vi "FRAS Module.vi"(0 "Cluster DATA TCL-TCL":T1={"SF_Mode"=enum."Repos", "SF_8x1_donnees(t)"=[], "SF_dark_monopixels"=[], "SF_lambdas"=[0.0, 0.0], "SF_matrice_ABCD"=[[0.0, 0.0, 0.0, 0.0], [0.0, 0.0, 0.0, 0.0], [0.0, 0.0, 0.0, 0.0], [0.0, 0.0, 0.0, 0.0], [0.0, 0.0, 0.0, 0.0], [0.0, 0.0, 0.0, 0.0], [0.0, 0.0, 0.0, 0.0], [0.0, 0.0, 0.0, 0.0]], "SF_ref"=0.0, "SF_ref_mode"=enum."Repos", "SF_ref_fichier"=0.0, "SF_OPD_estime"=[0.0, 0.0], "SF_OPD_mesure"=[[0.0, 0.0]], "SF_OPD_residus"=[[0.0, 0.0]], "SF_OPD_commande"=0.0, "SF_Intensites"=[0.0, 0.0], "SF_variables"=[], "SF_gain_int"=0.0, "FRAS_Mode"=enum."Repos", "FRAS_image_a"=[], "FRAS_image_b"=[], "FRAS_ref_images"=[], "FRAS_ref_mode"=enum."Repos", "FRAS_ref_fichier"=[], "FRAS_taille_images"=0, "FRAS_pourcentage_seuil"=0.0, "FRAS_CdG_calibration"=FALSE, "FRAS_CdG(t)"=[], "FRAS_CdG(t+1)"=[], "FRAS_CdG_residus"=[], "FRAS_gain_int"=0.0, "PERT_Mode"=enum."Repos", "PERT_saut_frange"=0, "PERT_offset"=[0.0, 0.0], "PERT_rep_PI"=0.0, "Nb Repetitions"=32, "PERT_booléens"=[], "coefficients"=[], "matrice_commande"=[], "Commande"=[], "Stop"=FALSE, "Nb boucles"=0, "Nb Retards"=0, "Nb Echantillons"=32, "Sauvegarde"=FALSE, "Nb Echantillons Cam"=32, "Increment Dark"=32, "SF_v_mesure"=[0.0, 0.0], "NbRepetConsig"=0, "DimConsignExt"=0, "ConsignExt"=[], "SF_Ref'"=0.0, "FRAS_Ref'"=[]}, 7 "Nb boucle":i32, 11 "entree d'erreur":errorcluster) -> (4 "Cluster DATA TCL-TCL":T1={"SF_Mode"=enum."Repos", "SF_8x1_donnees(t)"=[], "SF_dark_monopixels"=[], "SF_lambdas"=[0.0, 0.0], "SF_matrice_ABCD"=[[0.0, 0.0, 0.0, 0.0], [0.0, 0.0, 0.0, 0.0], [0.0, 0.0, 0.0, 0.0], [0.0, 0.0, 0.0, 0.0], [0.0, 0.0, 0.0, 0.0], [0.0, 0.0, 0.0, 0.0], [0.0, 0.0, 0.0, 0.0], [0.0, 0.0, 0.0, 0.0]], "SF_ref"=0.0, "SF_ref_mode"=enum."Repos", "SF_ref_fichier"=0.0, "SF_OPD_estime"=[0.0, 0.0], "SF_OPD_mesure"=[[0.0, 0.0]], "SF_OPD_residus"=[[0.0, 0.0]], "SF_OPD_commande"=0.0, "SF_Intensites"=[0.0, 0.0], "SF_variables"=[], "SF_gain_int"=0.0, "FRAS_Mode"=enum."Repos", "FRAS_image_a"=[], "FRAS_image_b"=[], "FRAS_ref_images"=[], "FRAS_ref_mode"=enum."Repos", "FRAS_ref_fichier"=[], "FRAS_taille_images"=0, "FRAS_pourcentage_seuil"=0.0, "FRAS_CdG_calibration"=FALSE, "FRAS_CdG(t)"=[], "FRAS_CdG(t+1)"=[], "FRAS_CdG_residus"=[], "FRAS_gain_int"=0.0, "PERT_Mode"=enum."Repos", "PERT_saut_frange"=0, "PERT_offset"=[0.0, 0.0], "PERT_rep_PI"=0.0, "Nb Repetitions"=32, "PERT_booléens"=[], "coefficients"=[], "matrice_commande"=[], "Commande"=[], "Stop"=FALSE, "Nb boucles"=0, "Nb Retards"=0, "Nb Echantillons"=32, "Sauvegarde"=FALSE, "Nb Echantillons Cam"=32, "Increment Dark"=32, "SF_v_mesure"=[0.0, 0.0], "NbRepetConsig"=0, "DimConsignExt"=0, "ConsignExt"=[], "SF_Ref'"=0.0, "FRAS_Ref'"=[]}, 15 "sortie d'erreur 2":errorcluster caption="sortie d'erreur")   [LabVIEW 2020]
uses:
  ACCROCHAGE/XPS_FGV.ctl
  DATACluster.ctl
panel:
  out "FRAS_ref_fichier":sgl[][](array[numeric])
  out "FRAS_Ref'":dbl[][](array[numeric])
  out "SF_Ref'":dbl
  out "ConsignExtSF":dbl[](array[numeric])
  out "ConsignExtFRAS":dbl[](array[numeric])
  out "cluster de sortie":cluster{"OPD":dbl, "W":dbl, "v_est":dbl}
  out "v2":dbl
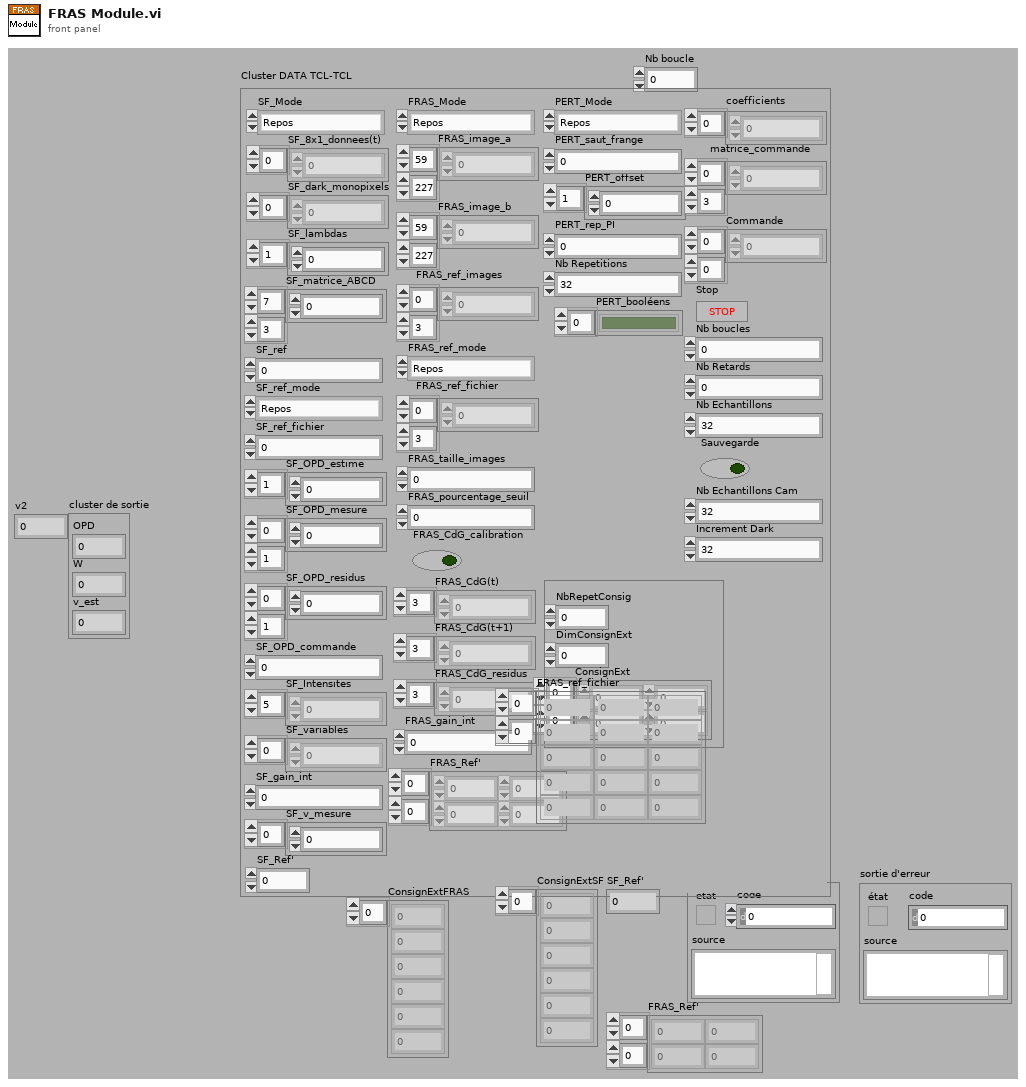
[diagram p1: front panel]
types:
  T1 = typedef "DATACluster.ctl" = cluster{"SF_Mode":enum16{"Repos", "Détection", "Acquisition", "Poursuite PID", "Poursuite Kalman", "Poursuite + contrôle"}, "SF_8x1_donnees(t)":dbl[], "SF_dark_monopixels":dbl[], "SF_lambdas":dbl[], "SF_matrice_ABCD":dbl[][], "SF_ref":dbl, "SF_ref_mode":enum16{"Repos", "Calibration", "Fichier"}, "SF_ref_fichier":dbl, "SF_OPD_estime":dbl[], "SF_OPD_mesure":dbl[][], "SF_OPD_residus":dbl[][], "SF_OPD_commande":dbl, "SF_Intensites":dbl[], "SF_variables":dbl[], "SF_gain_int":dbl, "FRAS_Mode":enum16{"Repos", "Détection", "Acquisition", "Poursuite", "Poursuite en a", "Poursuite en b"}, "FRAS_image_a":sgl[][], "FRAS_image_b":sgl[][], "FRAS_ref_images":sgl[][], "FRAS_ref_mode":enum16{"Repos", "Calibration", "Fichier"}, "FRAS_ref_fichier":sgl[][], "FRAS_taille_images":i32, "FRAS_pourcentage_seuil":sgl, "FRAS_CdG_calibration":bool, "FRAS_CdG(t)":dbl[], "FRAS_CdG(t+1)":dbl[], "FRAS_CdG_residus":dbl[], "FRAS_gain_int":dbl, "PERT_Mode":enum16{"Repos", "Calibration", "Fichier"}, "PERT_saut_frange":i8, "PERT_offset":dbl[], "PERT_rep_PI":dbl, "Nb Repetitions":i32, "PERT_booléens":bool[], "coefficients":dbl[], "matrice_commande":dbl[][], "Commande":dbl[][], "Stop":bool, "Nb boucles":i32, "Nb Retards":i16, "Nb Echantillons":i32, "Sauvegarde":bool, "Nb Echantillons Cam":i32, "Increment Dark":i32, "SF_v_mesure":dbl[], "NbRepetConsig":i32, "DimConsignExt":i32, "ConsignExt":dbl[][], "SF_Ref'":dbl, "FRAS_Ref'":dbl[][]}
  T2 = enum16{"Initialisation", "Acquisition", "Fermeture"}
  T3 = enum16{"Initialisation", "Calcul CdG a", "Calcul CdG b"}
  T4 = cluster{"Relative Target Position (units)":dbl, "Absolute Target Position (mm)":dbl}
  T5 = typedef "XPS_FGV.ctl" = enum16{"Init", "GroupKill", "GroupMotionEn", "GroupInit", "GroupHome", "ReadCurPos", "MoveAbs", "MoveRelatif", "JogEnable", "JogSet", "JogGet", "JogDisable", "ReadConfig", "GroupMotionDis", "Reboot", "Close"}
  T6 = cluster{"Velocity (units/s)":dbl, "Acceleration (units/s²)":dbl}
  T7 = typedef "IMAQ Image.ctl" = refnum<image>
  T8 = enum16{"Repos", "Détection", "Acquisition", "Poursuite", "Poursuite en a", "Poursuite en b"}
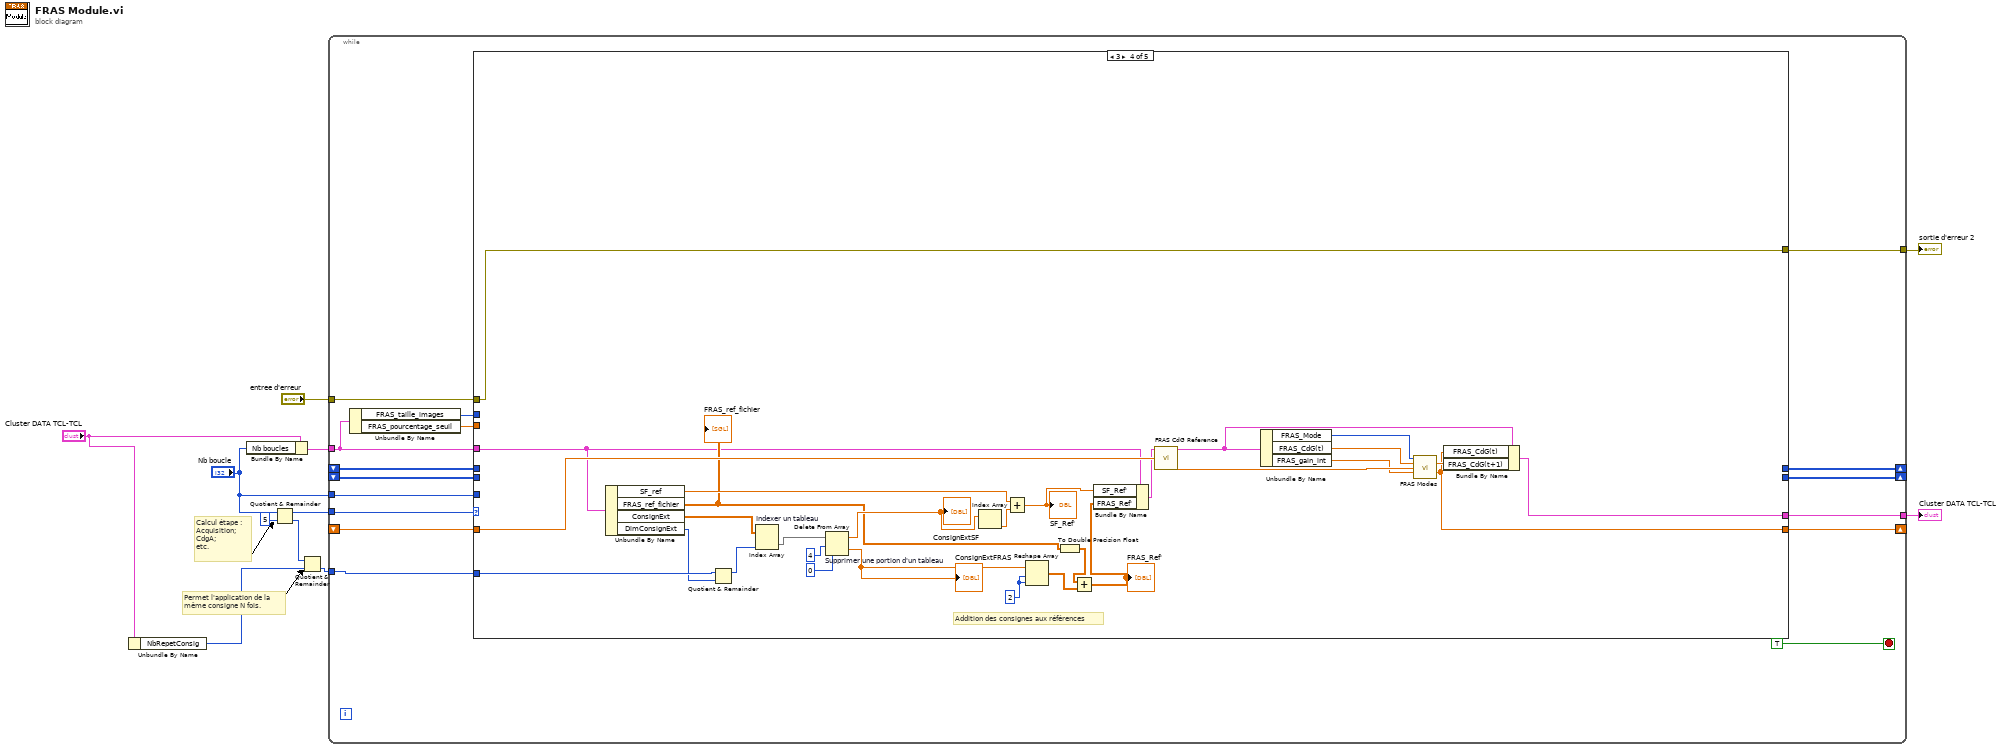
[diagram p0: block diagram]
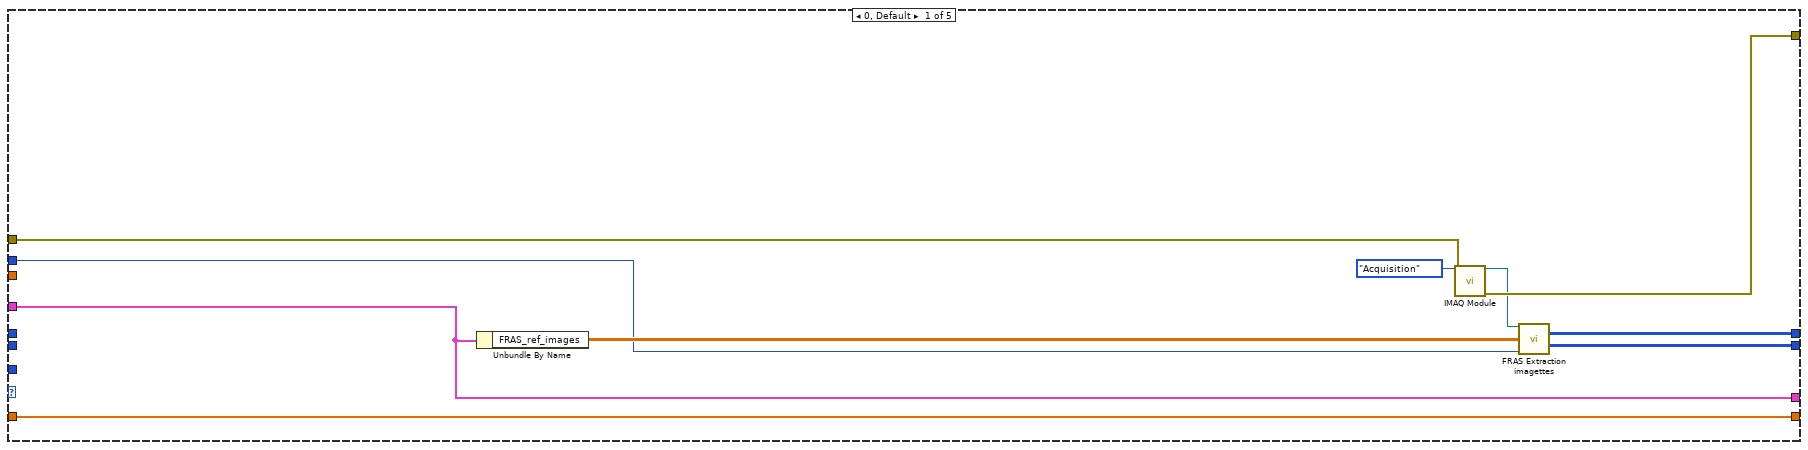
[diagram p2: hidden frame]
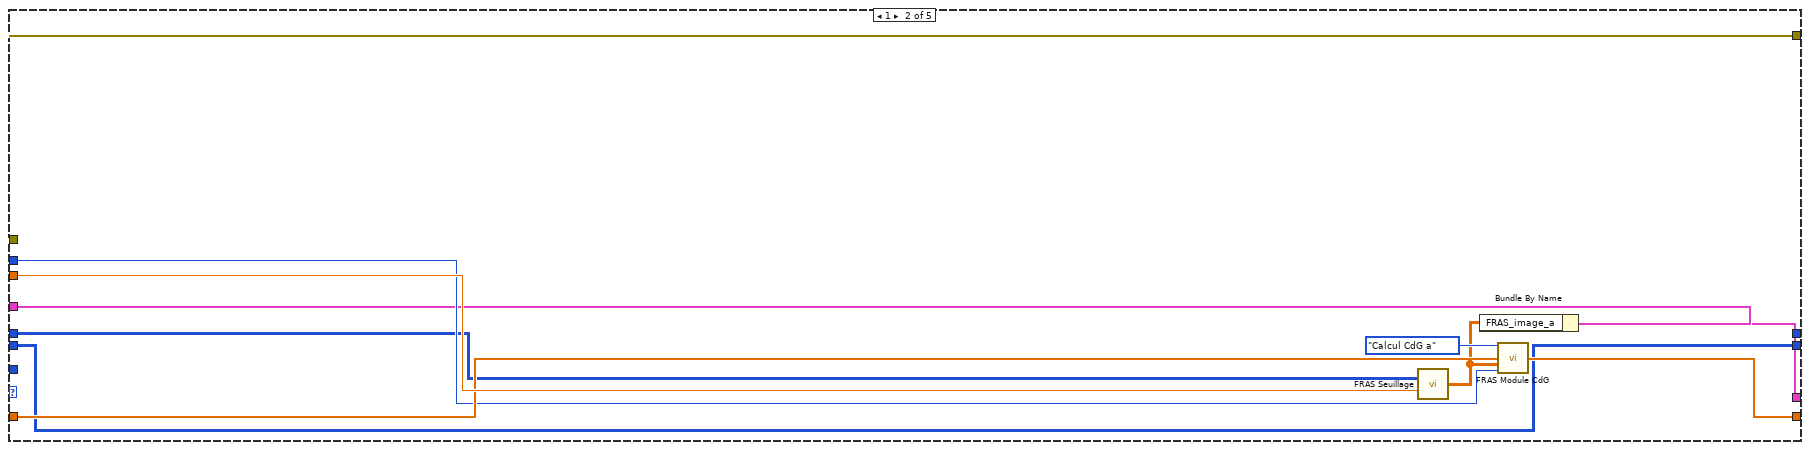
[diagram p3: hidden frame]
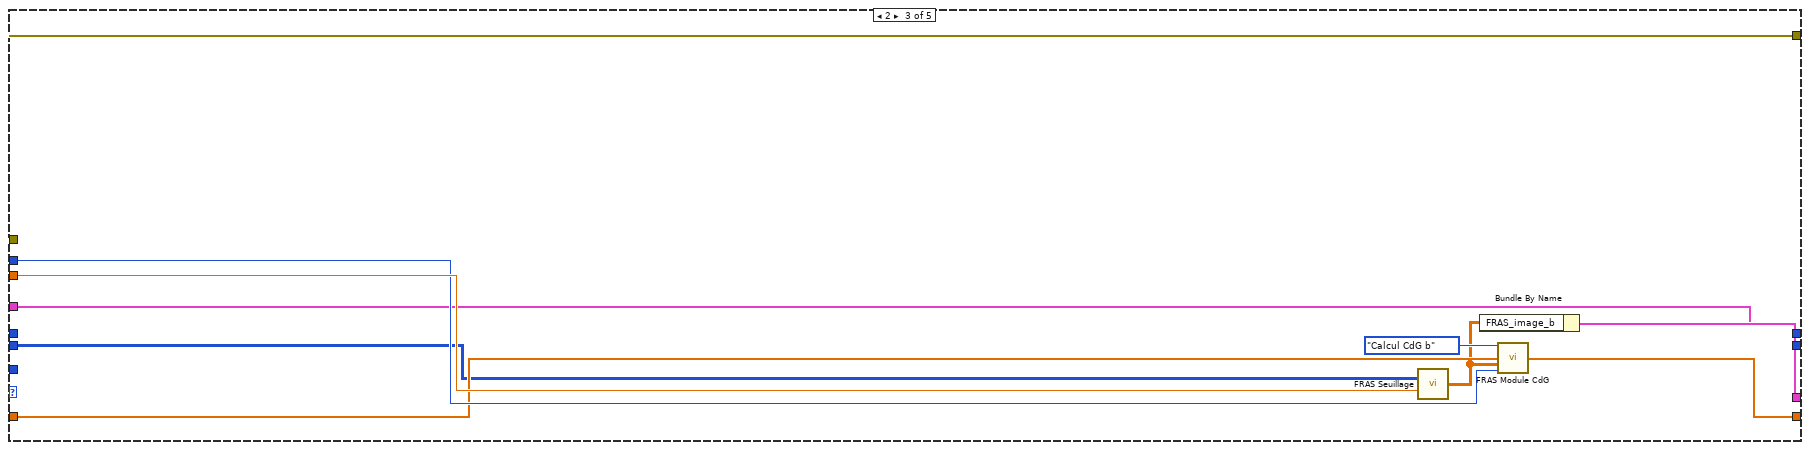
[diagram p4: hidden frame]
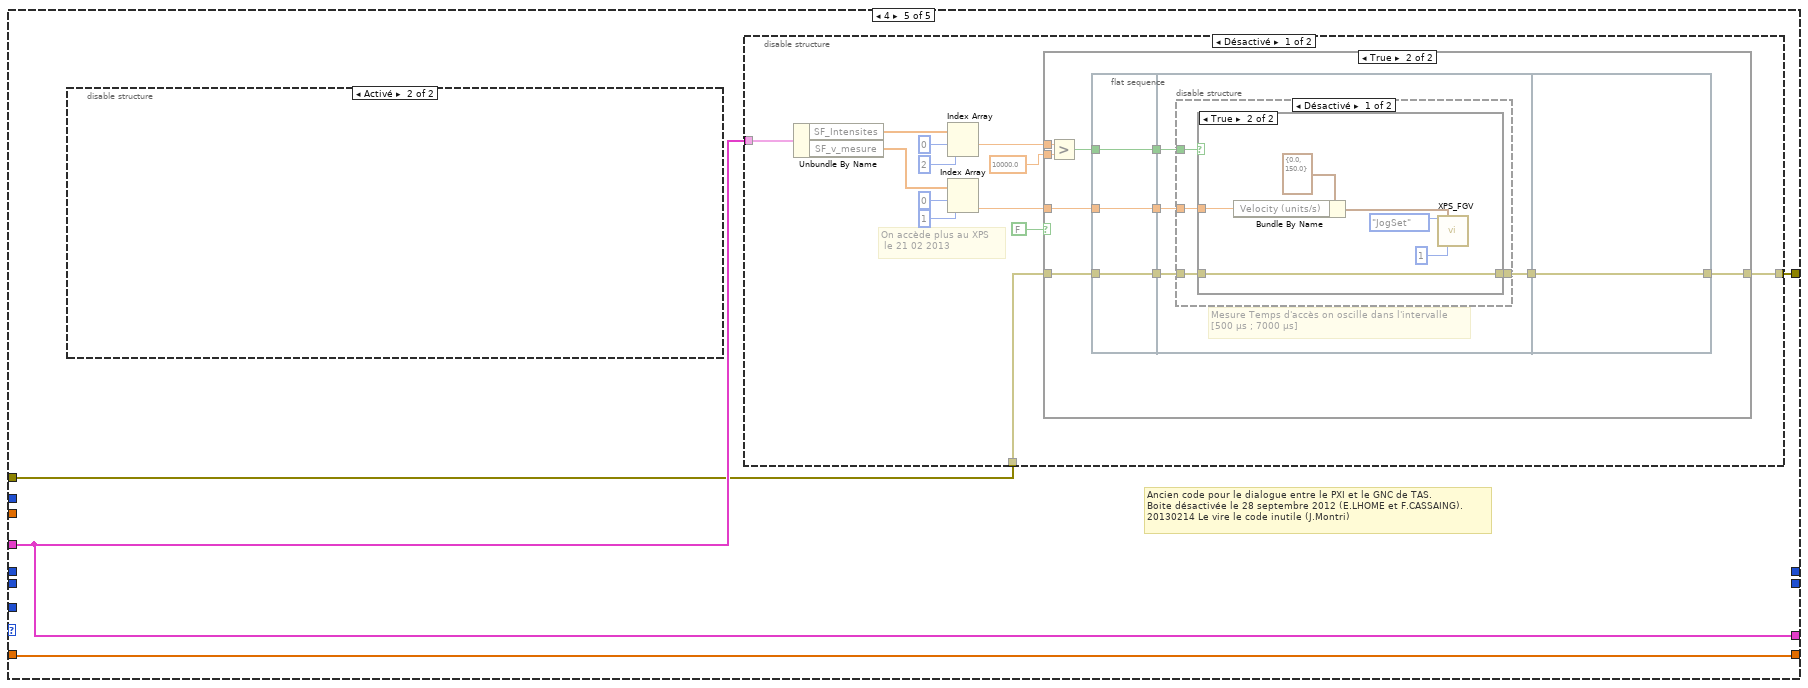
[diagram p5: hidden frame]
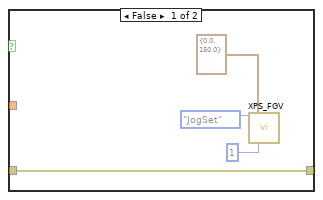
[diagram p7: hidden frame]
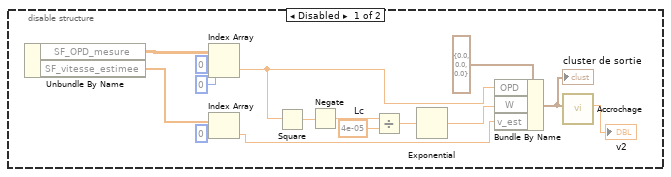
[diagram p10: hidden frame]
diagram:
  # "Permet l'application de la \nmême consigne N fois."
  # "Calcul étape : \nAcquisition; \nCdgA; \netc."
  n1 = Unbundle By Name("Cluster DATA TCL-TCL") -> ("NbRepetConsig"=w3:i32)
  n2 = Bundle By Name(cluster="Cluster DATA TCL-TCL", "Nb boucles"="Nb boucle") -> (w7:T1)
  n3 = Quotient & Remainder(x="Nb boucle", y=5) -> (x-y*floor(x/y)=w9:i32, floor(x/y)=w2:i32)
  n4 = Quotient & Remainder(x=w2, y=w3) -> (floor(x/y)=w1:i32)  [unwired: 1 out]
  n5 = while {
    tunnel: "entree d'erreur" -> [w22]
    tunnel: [w27] -> w10
    tunnel: w9 -> [w26]
    tunnel: w7 -> [w19]
    tunnel: [w16] -> w6
    shift-right: [w24] -> _
    shift-left: _ -> [w23]
    shift-right: [w21] -> _
    shift-left: _ -> [w20]
    shift-right: [w18] -> _
    shift-left: _ -> [w17]
    tunnel: "Nb boucle" -> [w15]
    tunnel: w1 -> [w12]
    stop <- TRUE stop-if-true
    n6 = Unbundle By Name(w19) -> ("FRAS_taille_images"=w14:i32, "FRAS_pourcentage_seuil"=w13:sgl)
    n7 = case shown="3" w26 {
      tunnel: [w36 w48 w58 w87 w89] -> w27
      tunnel: w22 -> [w37 w48 w58 w87 w88]
      tunnel: [w28 w41 w51 w78 w90] -> w16
      tunnel: w19 -> [w28 w42 w50 w61 w90]
      tunnel: [w30 w38 _ _ _] -> w24
      tunnel: w23 -> [_ w38 w52 _ _]
      tunnel: [w34 w45 w54 w79 w91] -> w21
      tunnel: w13 -> [_ w47 w57 _ _]
      tunnel: w20 -> [w34 w46 w55 w86 w91]
      tunnel: w14 -> [w31 w43 w56 _ _]
      tunnel: [w29 _ _ _ _] -> w18
      tunnel: w17 -> [_ w40 _ _ _]
      tunnel: w15 -> [_ _ _ _ _]
      tunnel: w12 -> [_ _ _ w77 _]
      frame 0, Default {
        n8 = Unbundle By Name(w28) -> ("FRAS_ref_images"=w33:sgl[][])
        n9 = call "IMAQ Module.vi"("Operation"=T2."Acquisition", "entree d'erreur"=w37) -> ("Image Out"=w32:T7, "sortie d'erreur"=w36:errorcluster)  [unwired: 12 out]
        n10 = call "FRAS Extraction imagettes.vi"("Image 2"=w32, "Coordonnées_Images"=w33, "Longueur du coté"=w31) -> ("Imagette1"=w29:i16[][], "Imagette2"=w30:i16[][])  [unwired: 11 out]
      }
      frame 1 {
        n11 = call "FRAS Seuillage.vi"("Imagette"=w40, "pourcentage max"=w47) -> ("Imagette seuillée"=w39:sgl[][])  [unwired: 13 out]
        n12 = Bundle By Name(cluster=w42, "FRAS_image_a"=w39) -> (w41:T1)
        n13 = call "FRAS Module CdG.vi"("Mode CdG"=T3."Calcul CdG a", "CdG in"=w46, "Imagette seuillée"=w39, "Largeur cote"=w43) -> ("CdG out"=w45:dbl[])  [unwired: 1 in, 10 out]
      }
      frame 2 {
        n14 = call "FRAS Seuillage.vi"("Imagette"=w52, "pourcentage max"=w57) -> ("Imagette seuillée"=w49:sgl[][])  [unwired: 13 out]
        n15 = Bundle By Name(cluster=w50, "FRAS_image_b"=w49) -> (w51:T1)
        n16 = call "FRAS Module CdG.vi"("Mode CdG"=T3."Calcul CdG b", "CdG in"=w55, "Imagette seuillée"=w49, "Largeur cote"=w56) -> ("CdG out"=w54:dbl[])  [unwired: 11 out]
      }
      frame 3 {
        w65 = 2 ("taille de la dimension")
        # "Addition des consignes aux références"
        n17 = Unbundle By Name(w61) -> ("SF_ref"=w68:dbl, "FRAS_ref_fichier"=w66:sgl[][], "ConsignExt"=w75:dbl[][], "DimConsignExt"=w76:i32)
        "FRAS_ref_fichier" <- w66
        n18 = Quotient & Remainder(x=w77, y=w76) -> (x-y*floor(x/y)=w74:i32)  [unwired: 1 out]
        n19 = Index Array "Indexer un tableau"(array=w75, index (col)=w74) -> (element=w73:dbl[])  [unwired: 1 in]
        n20 = Delete From Array "Supprimer une portion d'un tableau"(array=w73, length=4 ("indice"), index=0 ("longueur")) -> (deleted portion=w63:dbl[], array with subset deleted=w70:dbl[])
        "ConsignExtFRAS" <- w63
        "ConsignExtSF" <- w70
        n21 = Index Array(array=w70) -> (element=w69:dbl)  [unwired: 1 in]
        n22 = Add(x=w68, y=w69) -> (x+y=w60:dbl)
        "SF_Ref'" <- w60
        n23 = Reshape Array(w63, w65, w65) -> (w64:dbl[][])
        n24 = To Double Precision Float(number=w66) -> (double precision float=w67:dbl[][])
        n25 = Add(x=w67, y=w64) -> (x+y=w59:dbl[][])
        "FRAS_Ref'" <- w59
        n26 = Bundle By Name(cluster=w61, "SF_Ref'"=w60, "FRAS_Ref'"=w59) -> (w62:T1)
        n27 = call "FRAS CdG Reference.vi"("Cluster DATA TCL-TCL"=w62, "CdG(t)"=w86) -> ("Cluster DATA TCL-TCL"=w80:T1, "CdG res"=w85:dbl[])  [unwired: 12 out]
        n28 = Unbundle By Name(w80) -> ("FRAS_Mode"=w84:T8, "FRAS_CdG(t)"=w81:dbl[], "FRAS_gain_int"=w82:dbl)
        n29 = call "FRAS Modes.vi"("FRAS_Mode"=w84, "CdG(t)"=w81, "CdG res"=w85, "Gain_int"=w82) -> ("CdG(t+1)"=w83:dbl[], "CdG commande"=w79:dbl[])  [unwired: 10 out]
        n30 = Bundle By Name(cluster=w80, "FRAS_CdG(t)"=w79, "FRAS_CdG(t+1)"=w83) -> (w78:T1)
      }
      frame 4 {
        # "Ancien code pour le dialogue entre le PXI et le GNC de TAS.\nBoite désactivée le 28 septembre 2012 (E.LHOME et F.CASSAING).\n20130214 Le vire le code inutile (J.Montri)"
        n31 = disable-structure shown="Activé" {
          frame Disabled {
            w150 = 4e-05  # Lc
            n32 = Unbundle By Name() -> ("SF_OPD_mesure"=w144:dbl[][], "SF_vitesse_estimee"=w141:dbl[])  [unwired: 1 in]
            n33 = Index Array(array=w144, index (row)=0 ("indice (ligne)"), index (col)=0 ("indice désactivé (col)")) -> (element=w152:dbl)
            n34 = Index Array(array=w141, index=0 ("indice")) -> (element=w153:dbl)
            n35 = Square(x=w152) -> (x^2=w139:dbl)
            n36 = Negate(x=w139) -> (-x=w151:dbl)
            n37 = Divide(x=w151, y=w150) -> (x/y=w146:dbl)
            n38 = Exponential(1:w146) -> (0:w145:dbl)
            n39 = Bundle By Name(cluster=cluster{"OPD":dbl, "W":dbl, "v_est":dbl} {"OPD"=0.0, "W"=0.0, "v_est"=0.0} ("cluster d'entrée"), "OPD"=w152, "W"=w145, "v_est"=w153) -> (w148:cluster{"OPD":dbl, "W":dbl, "v_est":dbl})
            "cluster de sortie" <- w148
            n40 = call "Accrochage.vi"("cluster d'entrée"=w148) -> ("v2"=→"v2":dbl)  [unwired: 10 in]
          }
          frame Enabled {
          }
        }
        n41 = disable-structure shown="Désactivé" {
          disable-tunnel: w90 -> [w104 _]
          disable-tunnel: [w103 w138] -> w89
          disable-tunnel: w88 -> [w102 w138]
          frame Disabled {
            # "On accède plus au XPS \n le 21 02 2013"
            n42 = Unbundle By Name(w104) -> ("SF_Intensites"=w101:dbl[], "SF_v_mesure"=w95:dbl[])
            n43 = Index Array(array=w101, index #1=0 ("indice"), index #2=2 ("indice")) -> (element #1=w98:dbl)  [unwired: 1 out]
            n44 = Index Array(array=w95, index #1=0 ("indice"), index #2=1 ("indice")) -> (element #2=w93:dbl)  [unwired: 1 out]
            n45 = case shown="True" FALSE {
              tunnel: [w105 w111] -> w103
              tunnel: w102 -> [w105 w110]
              tunnel: w98 -> [_ w109]
              tunnel: 10000.0 ("y") -> [_ w108]
              tunnel: w93 -> [_ w106]
              frame False {
                # "On accède plus au XPS \n le 21 02 2013"
              }
              frame True {
                n46 = Greater?(x=w109, y=w108) -> (0:w107:bool)
                n47 = flat-sequence {
                  tunnel: w110 -> [w116]
                  tunnel: w106 -> [w117]
                  tunnel: w107 -> [w118]
                  tunnel: [w118] -> w115
                  tunnel: [w117] -> w114
                  tunnel: [w116] -> w113
                  tunnel: [w121] -> w112
                  tunnel: w115 -> [w122]
                  tunnel: w114 -> [w120]
                  tunnel: w113 -> [w119]
                  tunnel: [w137] -> w111
                  tunnel: w112 -> [w137]
                  frame #0 {
                  }
                  frame #1 {
                    # "Mesure Temps d'accès on oscille dans l'intervalle\n[500 µs ; 7000 µs]"
                    n48 = disable-structure shown="Désactivé" {
                      disable-tunnel: w122 -> [w126 _]
                      disable-tunnel: [w125 _] -> w121
                      disable-tunnel: w120 -> [w124 _]
                      disable-tunnel: w119 -> [w123 _]
                      frame Disabled {
                        n49 = case shown="True" w126 {
                          tunnel: w123 -> [w130 w134]
                          tunnel: [w130 w134] -> w125
                          tunnel: w124 -> [_ w131]
                          frame False {
                            n50 = call "XPS_FGV.vi"("Énum"=XPS_FGV."JogSet", "Group Jog parameters"=T4 {"Relative Target Position (units)"=0.0, "Absolute Target Position (mm)"=150.0} ("Cluster Data Pos In"), "NumPlatine"=1) -> ()  [unwired: 8 in, 5 out]
                          }
                          frame True {
                            n51 = Bundle By Name(cluster=T6 {"Velocity (units/s)"=0.0, "Acceleration (units/s²)"=150.0} ("Group Jog parameters"), "Velocity (units/s)"=w131) -> (w132:T6)
                            n52 = call "XPS_FGV.vi"("Énum"=XPS_FGV."JogSet", "Group Jog parameters"=w132, "NumPlatine"=1) -> ()  [unwired: 8 in, 5 out]
                          }
                        }
                      }
                      frame Enabled {
                      }
                    }
                  }
                  frame #2 {
                  }
                }
              }
            }
          }
          frame Enabled {
          }
        }
      }
    }
  }
  "sortie d'erreur 2" <- w10
  "Cluster DATA TCL-TCL" <- w6
